vi "testpet.vi"() -> ()   [LabVIEW 2016]
uses:
  Control/SafeMoveControl.ctl
panel:
  in  "Boolean":bool=TRUE
  in  "Move down 2":bool caption="Move"
  in  "Move up 2":bool caption="Move"
  in  "Tab Control":enum32{"Free", "Steps", "Total"}(tab)
  in  "Speed(µm)":dbl=500.0
  in  "Dis/Step(µm)":dbl=5.0
  in  "Step":i32=1
  in  "Dis/step(µm)":dbl=5.0
  in  "Speed(µm/s)":dbl=500.0
  in  "Speed(µm/s) 2":dbl=500.0
  in  "Total Distance(µm)":dbl=5.0
  in  "Dis/step(µm) 2":dbl=1.0
  in  "Pause":bool caption="Pause/resume"
  in  "Stop1":bool caption="Move"
  in  "Resume":bool caption="Pause/resume"
  in  "Stop3":bool caption="Move"
  in  "Move down":bool caption="Move"
  in  "Move up":bool caption="Move"
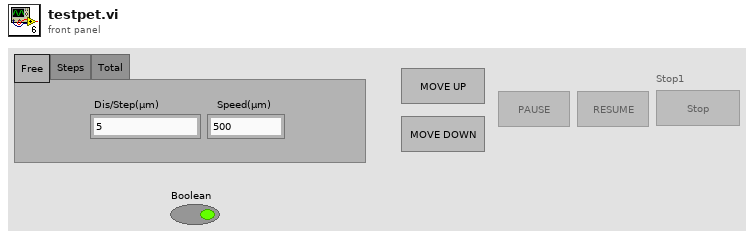
[diagram p1: front panel]
types:
  T1 = typedef "SafeMoveControl.ctl" = enum16{"Idle", "Pause", "Run2", "Run1"}
  T2 = enum8{"Enabled", "Disabled", "Disabled and Grayed Out"}
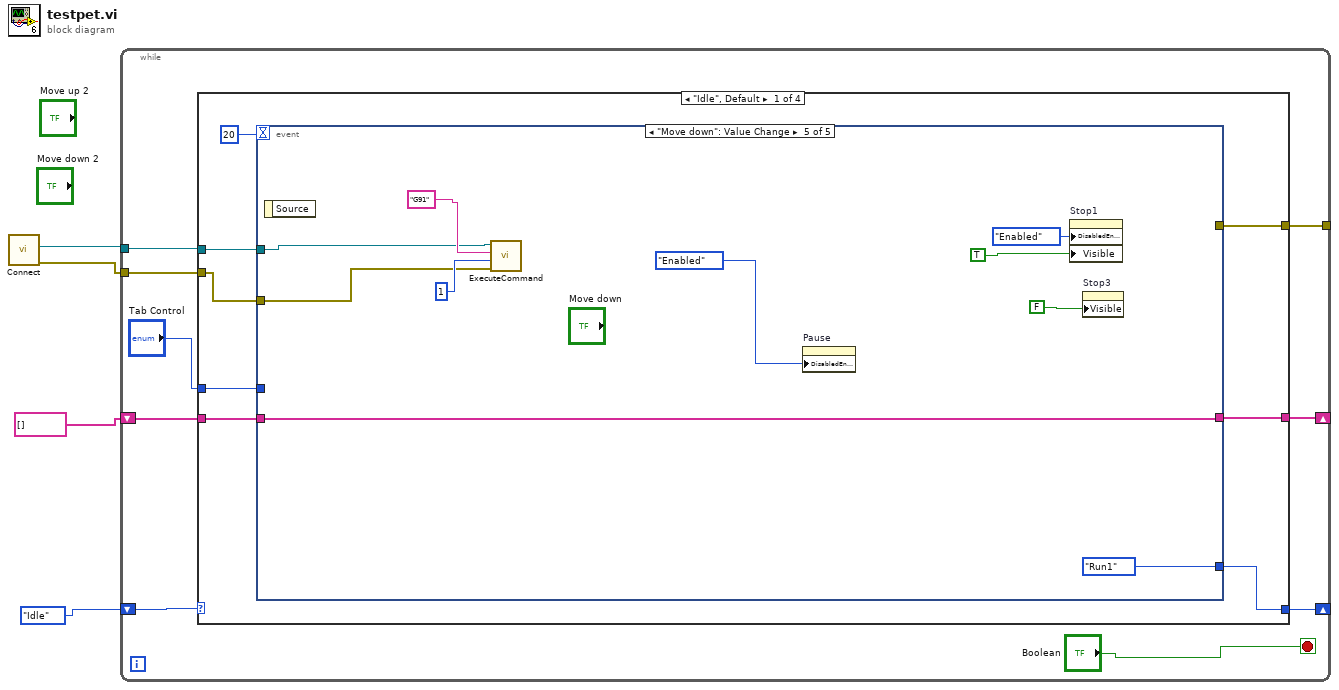
[diagram p0: block diagram]
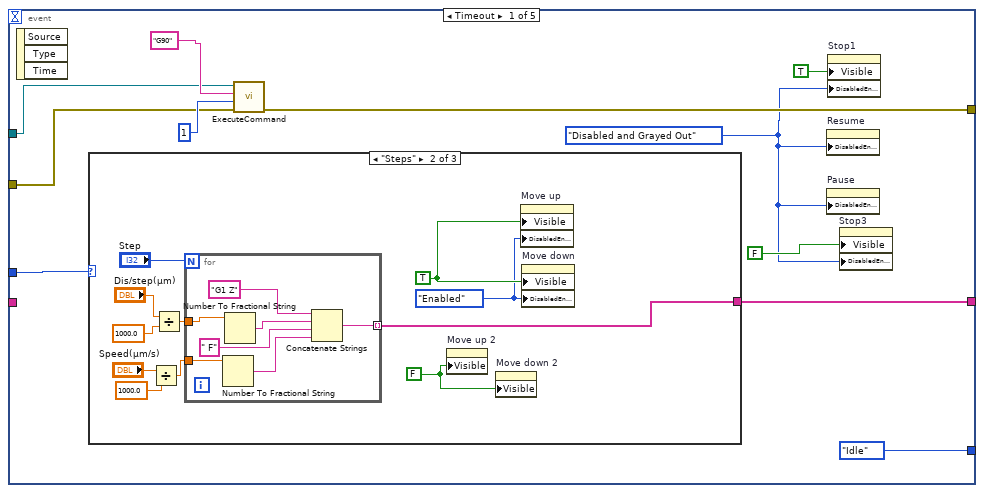
[diagram p2: hidden frame]
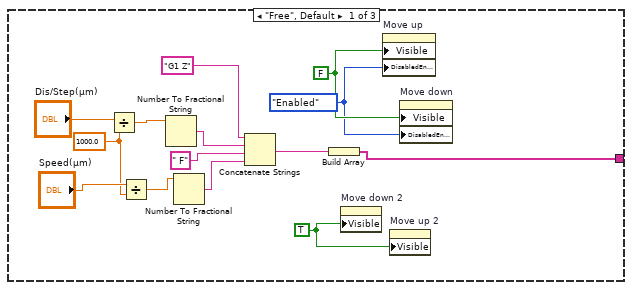
[diagram p3: hidden frame]
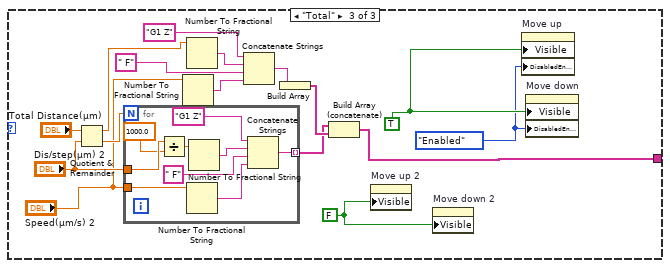
[diagram p4: hidden frame]
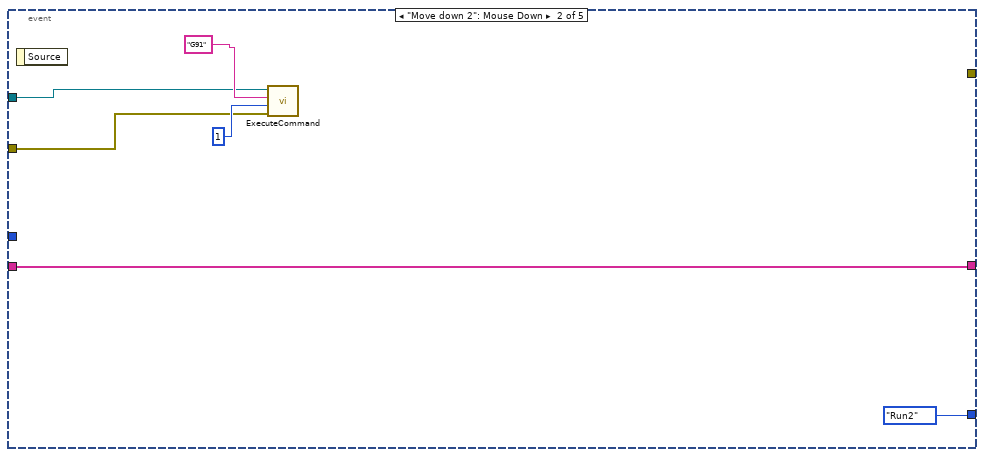
[diagram p5: hidden frame]
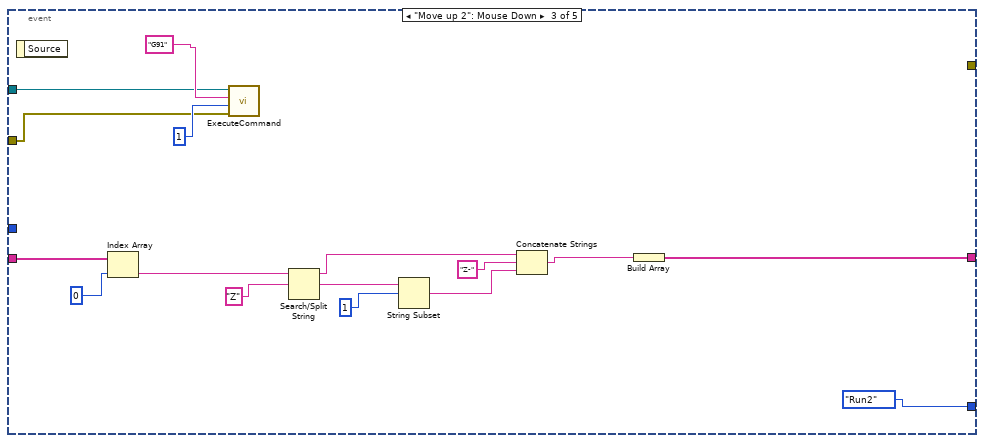
[diagram p6: hidden frame]
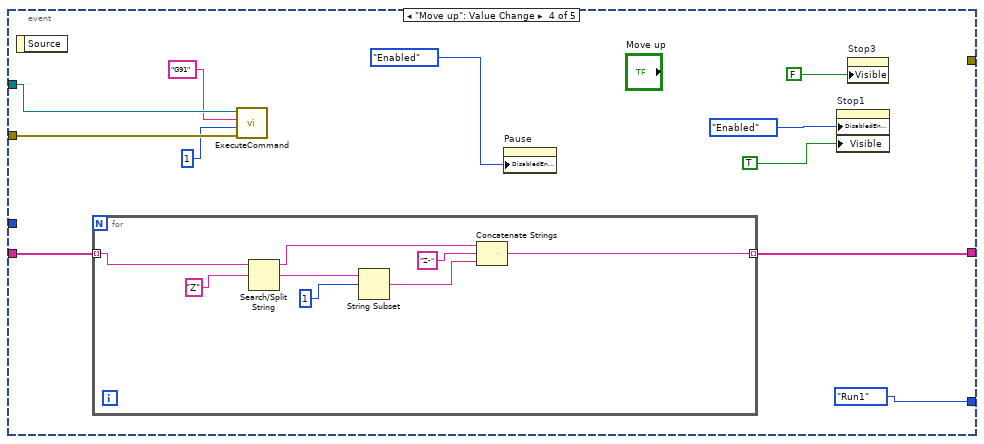
[diagram p7: hidden frame]
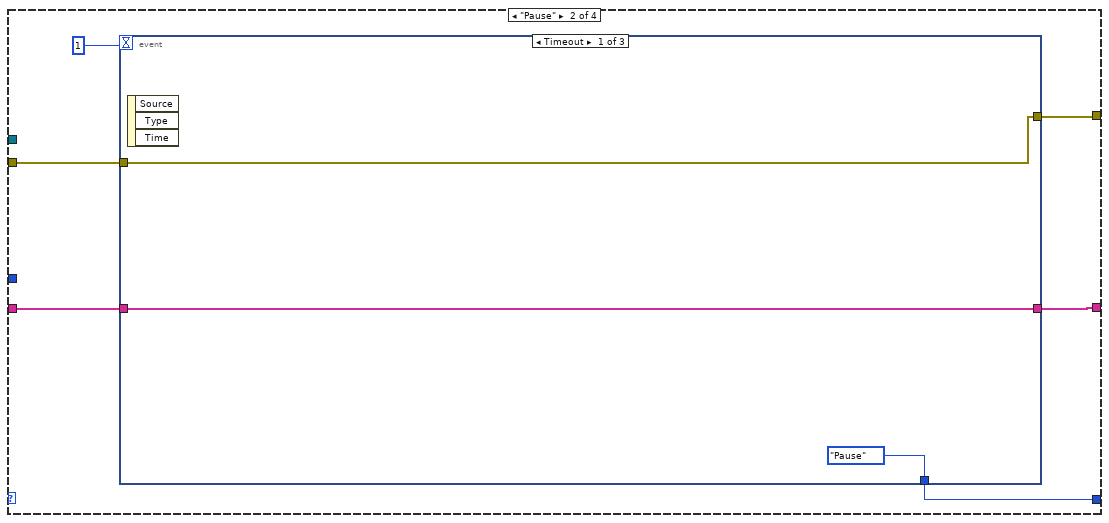
[diagram p8: hidden frame]
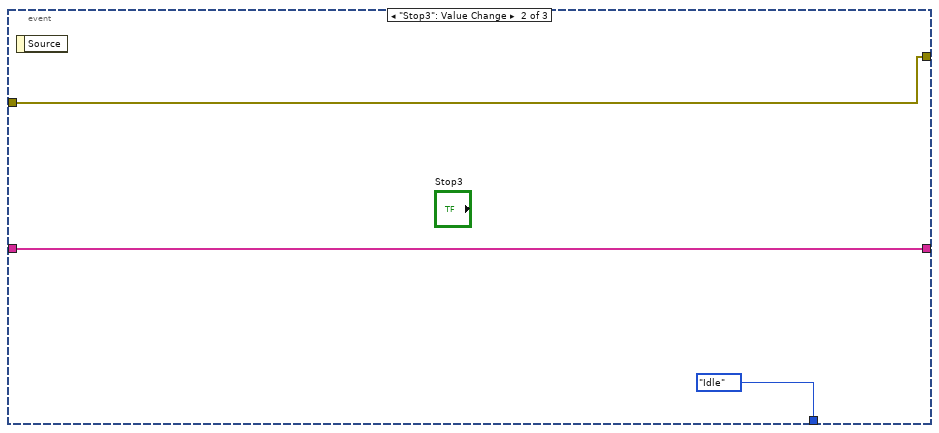
[diagram p9: hidden frame]
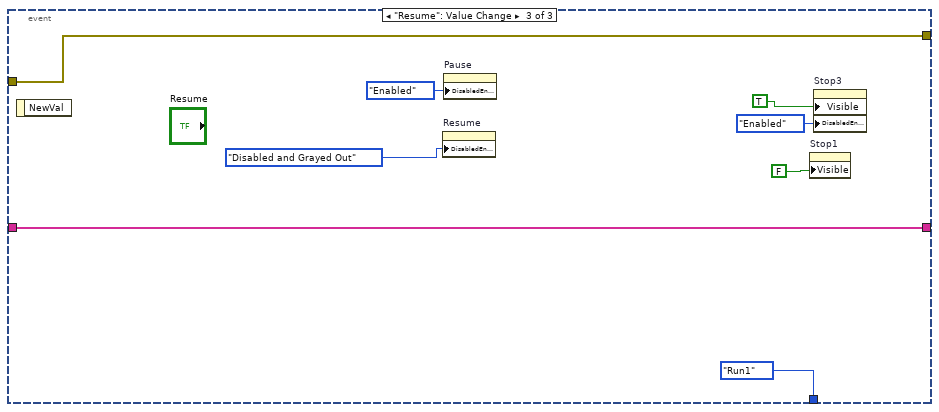
[diagram p10: hidden frame]
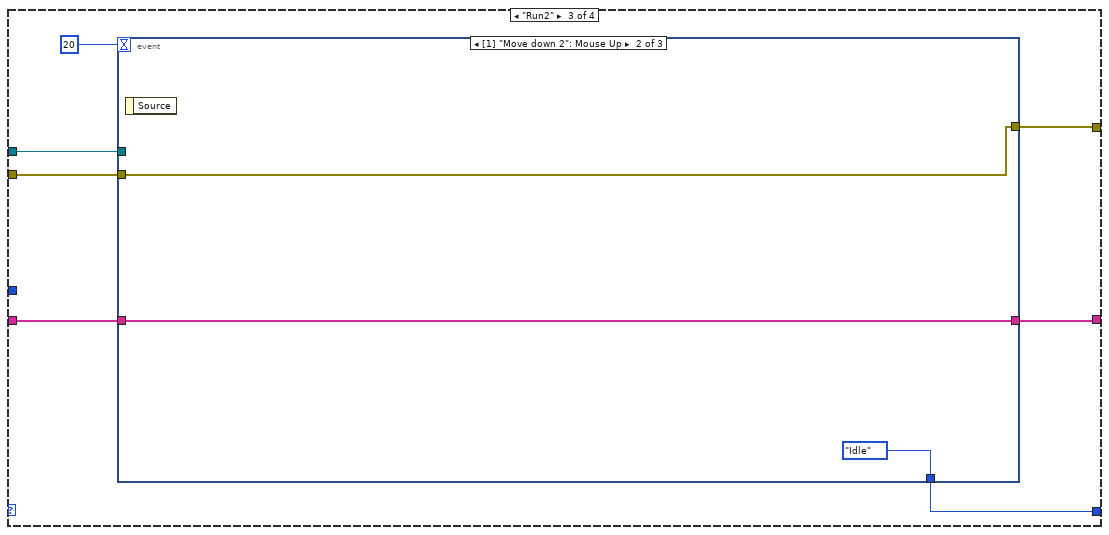
[diagram p11: hidden frame]
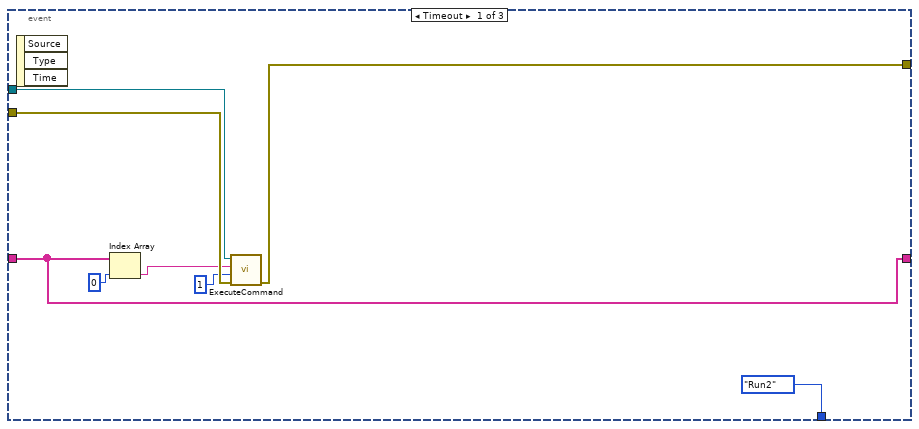
[diagram p12: hidden frame]
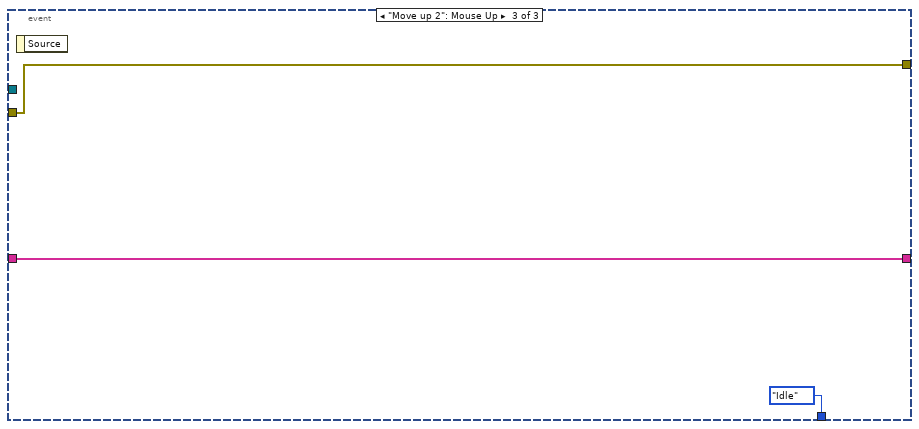
[diagram p13: hidden frame]
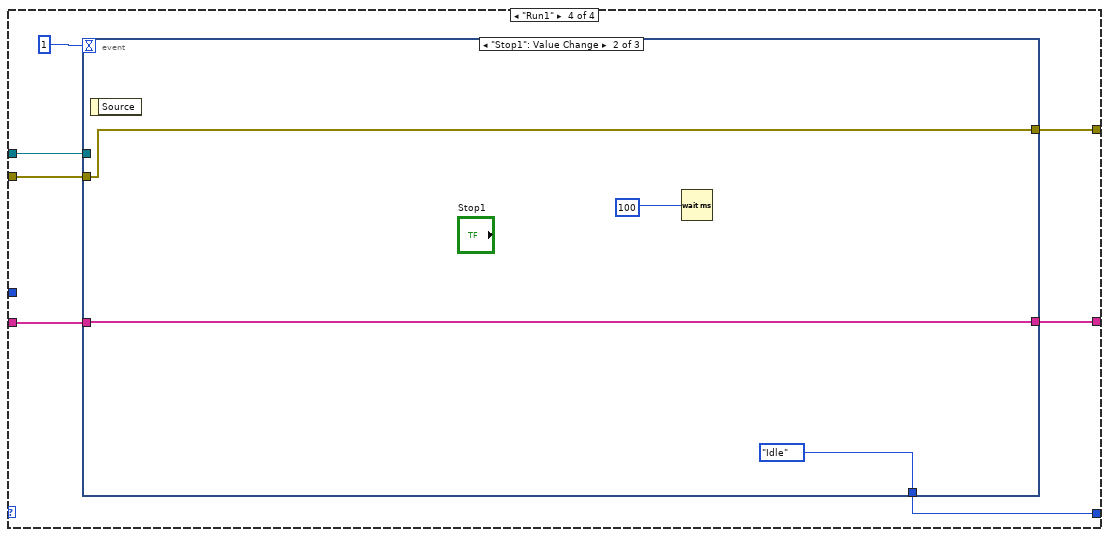
[diagram p14: hidden frame]
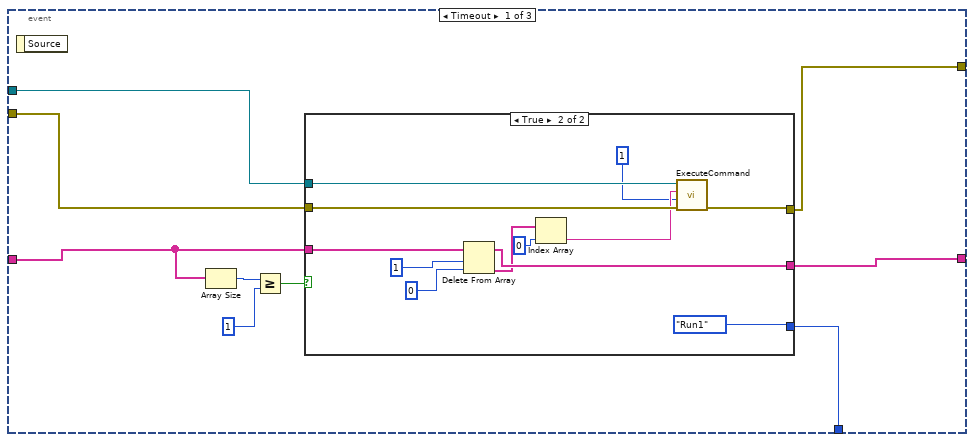
[diagram p15: hidden frame]
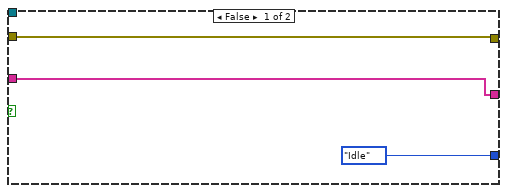
[diagram p16: hidden frame]
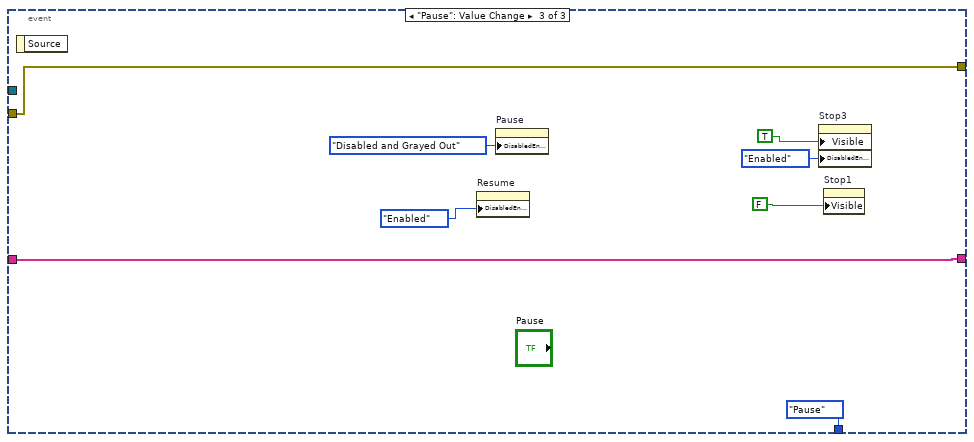
[diagram p17: hidden frame]
diagram:
  n1 = call "Connect.vi"() -> ("error out"=w1:errorcluster, "controller"=w2:refnum<k24>)  [unwired: 10 in]
  n2 = while {
    tunnel: w2 -> [w11]
    tunnel: w1 -> [w10]
    shift-right: [w12] -> _
    shift-left: SafeMoveControl."Idle" -> [w13]
    shift-right: [w8] -> _
    shift-left: string[] [] -> [w7]
    tunnel: [w6] -> _
    stop <- "Boolean" stop-if-true
    n3 = case shown="\"Idle\", Default" w13 {
      tunnel: [w21 w144 w165 w187] -> w12
      tunnel: w11 -> [w16 _ w164 w185]
      tunnel: w10 -> [w15 w143 w163 w186]
      tunnel: "Tab Control" -> [w20 _ _ _]
      tunnel: [w19 w145 w162 w183] -> w8
      tunnel: w7 -> [w18 w146 w166 w184]
      tunnel: [w14 w142 w161 w182] -> w6
      frame "Idle", Default {
        n4 = event shown="[4] \"Move down\": Value Change" {
          selector: _ -> [_ _ _ _ _]
          dyn-events: _ -> [_ _ _ _ _]
          timeout: 20 -> [_ _ _ _ _]
          tunnel: [enum16{"Idle"}."Idle" SafeMoveControl."Run2" SafeMoveControl."Run2" SafeMoveControl."Run1" SafeMoveControl."Run1"] -> w21
          tunnel: w20 -> [w31 _ _ _ _]
          tunnel: [w30 w94 w100 w119 w138] -> w19
          tunnel: w18 -> [_ w94 w104 w120 w138]
          tunnel: w16 -> [w27 w91 w97 w118 w135]
          tunnel: w15 -> [w26 w90 w96 w117 w134]
          tunnel: [w25 _ _ _ _] -> w14
          event Timeout {
            w22 = T2."Disabled and Grayed Out" ("Disabled")
            n5 = event-data() -> ()  [unwired: 1 in, 3 out]
            n6 = case shown="\"Steps\"" w31 {
              tunnel: [w39 w56 w68] -> w30
              frame "Free", Default {
                w33 = T2."Enabled" ("Disabled")
                w34 = 1000.0
                w45 = TRUE
                w46 = FALSE
                n7 = Divide(x="Dis/Step(µm)", y=w34) -> (x/y=w37:dbl)
                n8 = Divide(x="Speed(µm)", y=w34) -> (x/y=w36:dbl)
                n9 = Number To Fractional String(number=w37) -> (F-format string=w43:string)  [unwired: 3 in]
                n10 = Number To Fractional String(number=w36) -> (F-format string=w41:string)  [unwired: 3 in]
                n11 = Concatenate Strings("G1 Z", w43, " F", w41) -> (w40:string)
                n12 = Build Array(w40) -> (w39:string[])
                n13 = property on="Move down 2" class="Bool (strict)"("Visible"=w45) -> ()  [unwired: 2 in, 2 out]
                n14 = property on="Move up" class="Bool"("Visible"=w46, "DisabledEnum"=w33) -> ()  [unwired: 2 in, 2 out]
                n15 = property on="Move up 2" class="Bool (strict)"("Visible"=w45) -> ()  [unwired: 2 in, 2 out]
                n16 = property on="Move down" class="Bool"("Visible"=w46, "DisabledEnum"=w33) -> ()  [unwired: 2 in, 2 out]
              }
              frame "Steps" {
                w47 = T2."Enabled" ("Disabled")
                w51 = FALSE
                w52 = TRUE
                n17 = Divide(x="Speed(µm/s)", y=1000.0) -> (x/y=w53:dbl)
                n18 = Divide(x="Dis/step(µm)", y=1000.0) -> (x/y=w48:dbl)
                n19 = for {
                  N: "Step" -> [_]
                  tunnel: w53 -> [w64]
                  tunnel: [w59] -> w56 mode=indexing
                  tunnel: w48 -> [w58]
                  n20 = Number To Fractional String(number=w64) -> (F-format string=w60:string)  [unwired: 3 in]
                  n21 = Number To Fractional String(number=w58) -> (F-format string=w63:string)  [unwired: 3 in]
                  n22 = Concatenate Strings("G1 Z", w63, " F", w60) -> (w59:string)
                }
                n23 = property on="Move up 2" class="Bool (strict)"("Visible"=w51) -> ()  [unwired: 2 in, 2 out]
                n24 = property on="Move down 2" class="Bool (strict)"("Visible"=w51) -> ()  [unwired: 2 in, 2 out]
                n25 = property on="Move up" class="Bool"("Visible"=w52, "DisabledEnum"=w47) -> ()  [unwired: 2 in, 2 out]
                n26 = property on="Move down" class="Bool"("Visible"=w52, "DisabledEnum"=w47) -> ()  [unwired: 2 in, 2 out]
              }
              frame "Total" {
                w65 = T2."Enabled" ("Disabled")
                w79 = FALSE
                w80 = TRUE
                n27 = Quotient & Remainder(x="Total Distance(µm)", y="Dis/step(µm) 2") -> (x-y*floor(x/y)=w70:dbl, floor(x/y)=w77:dbl)
                n28 = for {
                  N: w77 -> [_]
                  tunnel: "Speed(µm/s) 2" -> [w86]
                  tunnel: "Dis/step(µm) 2" -> [w82]
                  tunnel: [w84] -> w66 mode=indexing
                  n29 = Divide(x=w82, y=1000.0) -> (x/y=w83:dbl)
                  n30 = Number To Fractional String(number=w86) -> (F-format string=w85:string)  [unwired: 3 in]
                  n31 = Number To Fractional String(number=w83) -> (F-format string=w89:string)  [unwired: 3 in]
                  n32 = Concatenate Strings("G1 Z", w89, " F", w85) -> (w84:string)
                }
                n33 = Number To Fractional String(number="Speed(µm/s) 2") -> (F-format string=w73:string)  [unwired: 3 in]
                n34 = Number To Fractional String(number=w70) -> (F-format string=w72:string)  [unwired: 3 in]
                n35 = Concatenate Strings("G1 Z", w72, " F", w73) -> (w75:string)
                n36 = Build Array(w75) -> (w67:string[])
                n37 = Build Array (concatenate)(w66, w67) -> (w68:string[])
                n38 = property on="Move up 2" class="Bool (strict)"("Visible"=w79) -> ()  [unwired: 2 in, 2 out]
                n39 = property on="Move down 2" class="Bool (strict)"("Visible"=w79) -> ()  [unwired: 2 in, 2 out]
                n40 = property on="Move up" class="Bool"("Visible"=w80, "DisabledEnum"=w65) -> ()  [unwired: 2 in, 2 out]
                n41 = property on="Move down" class="Bool"("Visible"=w80, "DisabledEnum"=w65) -> ()  [unwired: 2 in, 2 out]
              }
            }
            n42 = call "ExecuteCommand.vi"("error in (no error)"=w26, "taskId"=1, "Command Code"="G90", "controller in"=w27) -> ("error out"=w25:errorcluster)  [unwired: 5 in, 2 out]
            n43 = property on="Resume" class="Bool"("DisabledEnum"=w22) -> ()  [unwired: 2 in, 2 out]
            n44 = property on="Pause" class="Bool"("DisabledEnum"=w22) -> ()  [unwired: 2 in, 2 out]
            n45 = property on="Stop1" class="Bool (strict)"("Visible"=TRUE, "DisabledEnum"=w22) -> ()  [unwired: 2 in, 2 out]
            n46 = property on="Stop3" class="Bool (strict)"("Visible"=FALSE, "DisabledEnum"=w22) -> ()  [unwired: 2 in, 2 out]
          }
          event "Move down 2": Mouse Down {
            n47 = event-data() -> ()  [unwired: 1 in, 1 out]
            n48 = call "ExecuteCommand.vi"("error in (no error)"=w90, "taskId"=1, "Command Code"="G91", "controller in"=w91) -> ()  [unwired: 5 in, 3 out]
          }
          event "Move up 2": Mouse Down {
            n49 = event-data() -> ()  [unwired: 1 in, 1 out]
            n50 = Index Array(array=w104, index=0) -> (element=w102:string)
            n51 = call "ExecuteCommand.vi"("error in (no error)"=w96, "taskId"=1, "Command Code"="G91", "controller in"=w97) -> ()  [unwired: 5 in, 3 out]
            n52 = Search/Split String(string=w102, search string/char (-)="Z") -> (substring before match=w107:string, match + rest of string=w109:string)  [unwired: 1 in, 1 out]
            n53 = String Subset(string=w109, offset (0)=1) -> (substring=w105:string)  [unwired: 1 in]
            n54 = Concatenate Strings(w107, "Z-", w105) -> (w101:string)
            n55 = Build Array(w101) -> (w100:string[])
          }
          event "Move up": Value Change {
            n56 = event-data() -> ()  [unwired: 1 in, 1 out]
            n57 = for {
              tunnel: w120 -> [w130] mode=indexing
              tunnel: [w123] -> w119 mode=indexing
              n58 = Search/Split String(string=w130, search string/char (-)="Z") -> (substring before match=w126:string, match + rest of string=w128:string)  [unwired: 1 in, 1 out]
              n59 = String Subset(string=w128, offset (0)=1) -> (substring=w124:string)  [unwired: 1 in]
              n60 = Concatenate Strings(w126, "Z-", w124) -> (w123:string)
            }
            n61 = call "ExecuteCommand.vi"("error in (no error)"=w117, "taskId"=1, "Command Code"="G91", "controller in"=w118) -> ()  [unwired: 5 in, 3 out]
            n62 = property on="Pause" class="Bool"("DisabledEnum"=T2."Enabled" ("Disabled")) -> ()  [unwired: 2 in, 2 out]
            n63 = property on="Stop1" class="Bool (strict)"("DisabledEnum"=T2."Enabled" ("Disabled"), "Visible"=TRUE) -> ()  [unwired: 2 in, 2 out]
            n64 = property on="Stop3" class="Bool (strict)"("Visible"=FALSE) -> ()  [unwired: 2 in, 2 out]
          }
          event "Move down": Value Change {
            n65 = event-data() -> ()  [unwired: 1 in, 1 out]
            n66 = call "ExecuteCommand.vi"("error in (no error)"=w134, "taskId"=1, "Command Code"="G91", "controller in"=w135) -> ()  [unwired: 5 in, 3 out]
            n67 = property on="Pause" class="Bool"("DisabledEnum"=T2."Enabled" ("Disabled")) -> ()  [unwired: 2 in, 2 out]
            n68 = property on="Stop1" class="Bool (strict)"("DisabledEnum"=T2."Enabled" ("Disabled"), "Visible"=TRUE) -> ()  [unwired: 2 in, 2 out]
            n69 = property on="Stop3" class="Bool (strict)"("Visible"=FALSE) -> ()  [unwired: 2 in, 2 out]
          }
        }
      }
      frame "Pause" {
        n70 = event shown="[0] Timeout" {
          selector: _ -> [_ _ _]
          dyn-events: _ -> [_ _ _]
          timeout: 1 -> [_ _ _]
          tunnel: w146 -> [w149 w151 w160]
          tunnel: [w149 w151 w160] -> w145
          tunnel: [SafeMoveControl."Pause" SafeMoveControl."Idle" SafeMoveControl."Run1"] -> w144
          tunnel: w143 -> [w147 w152 w156]
          tunnel: [w147 w152 w156] -> w142
          event Timeout {
            n71 = event-data() -> ()  [unwired: 1 in, 3 out]
          }
          event "Stop3": Value Change {
            n72 = event-data() -> ()  [unwired: 1 in, 1 out]
          }
          event "Resume": Value Change {
            n73 = event-data() -> ()  [unwired: 1 in, 1 out]
            n74 = property on="Resume" class="Bool"("DisabledEnum"=T2."Disabled and Grayed Out" ("Disabled")) -> ()  [unwired: 2 in, 2 out]
            n75 = property on="Pause" class="Bool"("DisabledEnum"=T2."Enabled" ("Disabled")) -> ()  [unwired: 2 in, 2 out]
            n76 = property on="Stop1" class="Bool (strict)"("Visible"=FALSE) -> ()  [unwired: 2 in, 2 out]
            n77 = property on="Stop3" class="Bool (strict)"("Visible"=TRUE, "DisabledEnum"=T2."Enabled" ("Disabled")) -> ()  [unwired: 2 in, 2 out]
          }
        }
      }
      frame "Run2" {
        n78 = event shown="[1] \"Move down 2\": Mouse Up" {
          selector: _ -> [_ _ _]
          dyn-events: _ -> [_ _ _]
          timeout: 20 -> [_ _ _]
          tunnel: w166 -> [w170 w177 w180]
          tunnel: [SafeMoveControl."Run2" SafeMoveControl."Idle" SafeMoveControl."Idle"] -> w165
          tunnel: w164 -> [w174 _ _]
          tunnel: w163 -> [w173 w176 w179]
          tunnel: [w170 w177 w180] -> w162
          tunnel: [w168 w176 w179] -> w161
          event Timeout {
            n79 = event-data() -> ()  [unwired: 1 in, 3 out]
            n80 = Index Array(array=w170, index=0) -> (element=w172:string)
            n81 = call "ExecuteCommand.vi"("error in (no error)"=w173, "taskId"=1, "Command Code"=w172, "controller in"=w174) -> ("error out"=w168:errorcluster)  [unwired: 5 in, 2 out]
          }
          event "Move down 2": Mouse Up {
            n82 = event-data() -> ()  [unwired: 1 in, 1 out]
          }
          event "Move up 2": Mouse Up {
            n83 = event-data() -> ()  [unwired: 1 in, 1 out]
          }
        }
      }
      frame "Run1" {
        n84 = event shown="[1] \"Stop1\": Value Change" {
          selector: _ -> [_ _ _]
          dyn-events: _ -> [_ _ _]
          timeout: 1 -> [_ _ _]
          tunnel: [w190 SafeMoveControl."Idle" SafeMoveControl."Pause"] -> w187
          tunnel: w186 -> [w196 w215 w220]
          tunnel: w185 -> [w197 _ _]
          tunnel: w184 -> [w194 w216 w223]
          tunnel: [w195 w216 w223] -> w183
          tunnel: [w189 w215 w220] -> w182
          event Timeout {
            n85 = event-data() -> ()  [unwired: 1 in, 1 out]
            n86 = Array Size(array=w194) -> (size(s)=w193:i32)
            n87 = Greater Or Equal?(x=w193, y=1) -> (x >= y?=w191:bool)
            n88 = case shown="True" w191 {
              tunnel: w197 -> [_ w212]
              tunnel: w196 -> [w198 w211]
              tunnel: [w200 w203] -> w195
              tunnel: w194 -> [w200 w205]
              tunnel: [SafeMoveControl."Idle" SafeMoveControl."Run1"] -> w190
              tunnel: [w198 w201] -> w189
              frame False {
              }
              frame True {
                n89 = Delete From Array(array=w205, length=1, index=0) -> (deleted portion=w202:string[], array with subset deleted=w203:string[])
                n90 = Index Array(array=w202, index=0) -> (element=w208:string)
                n91 = call "ExecuteCommand.vi"("error in (no error)"=w211, "taskId"=1, "Command Code"=w208, "controller in"=w212) -> ("error out"=w201:errorcluster)  [unwired: 5 in, 2 out]
              }
            }
          }
          event "Stop1": Value Change {
            n92 = event-data() -> ()  [unwired: 1 in, 1 out]
            n93 = Wait (ms)(milliseconds to wait=100) -> ()  [unwired: 1 out]
          }
          event "Pause": Value Change {
            n94 = event-data() -> ()  [unwired: 1 in, 1 out]
            n95 = property on="Resume" class="Bool"("DisabledEnum"=T2."Enabled" ("Disabled")) -> ()  [unwired: 2 in, 2 out]
            n96 = property on="Pause" class="Bool"("DisabledEnum"=T2."Disabled and Grayed Out" ("Disabled")) -> ()  [unwired: 2 in, 2 out]
            n97 = property on="Stop3" class="Bool (strict)"("Visible"=TRUE, "DisabledEnum"=T2."Enabled" ("Disabled")) -> ()  [unwired: 2 in, 2 out]
            n98 = property on="Stop1" class="Bool (strict)"("Visible"=FALSE) -> ()  [unwired: 2 in, 2 out]
          }
        }
      }
    }
  }
